vi "Connect.vi"(8 "error in (no error)":errorcluster, 9 "timeout":i32=-1, 11 "TCP Stream Listener in":refnum<class "TCP Stream Listener.lvclass">) -> (0 "error out":errorcluster, 3 "TCP Stream Listener out":refnum<class "TCP Stream Listener.lvclass">)   [LabVIEW 2020, in "TCP Stream Listener.lvclass"]
doc: "This method waits for a remote connection from a TCP/IP Stream Initiator."
uses:
  TCP Stream Listener.lvclass
  G:/Utilisateurs/hugofroylan.aragon/Documents/PyCharm/neuro/labview/Nested Endpoint Actors/Protocols/TCP Strategy/TCP Stream/TCP Stream.lvclass
  TCP Stream/TCP Stream.lvclass/TCP Stream.ctl
  TCP Stream Listener.lvclass/TCP Stream Listener.ctl
  TCP Stream/TCP Stream.lvclass
  libc.so.6
  C:/Windows/System32/ws2_32.dll
panel:
  out "return 2":i32
  out "return":i32
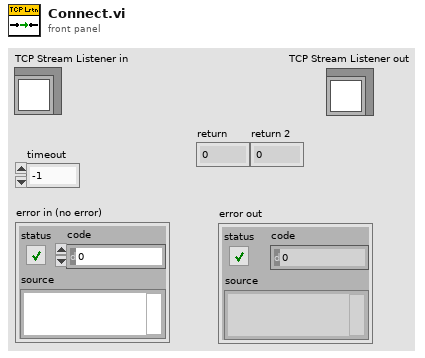
[diagram p1: front panel]
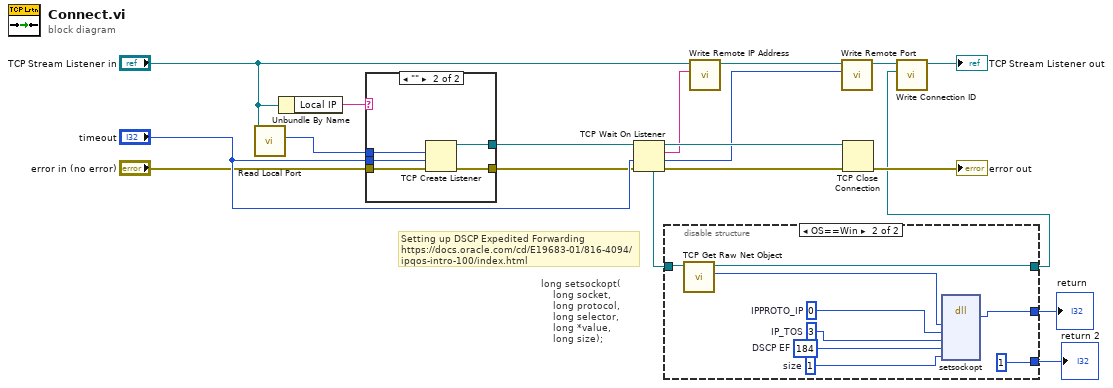
[diagram p0: block diagram]
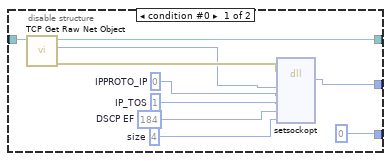
[diagram p2: hidden frame]
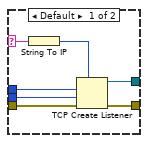
[diagram p3: hidden frame]
diagram:
  # "long setsockopt(\n    long socket,\n    long protocol,\n    long selector,\n    long *value,\n    long size);"
  # "Setting up DSCP Expedited Forwarding\nhttps://docs.oracle.com/cd/E19683-01/816-4094/ipqos-intro-100/index.html"
  n1 = call "Read Local Port.vi"("TCP Stream in"="TCP Stream Listener in") -> ("local port"=w15:u16)  [unwired: 10 in]
  n2 = Unbundle By Name("TCP Stream Listener in") -> ("Local IP"=w10:string)
  n3 = case shown="\"\"" w10 {
    selector: w10 -> [w21 _]
    tunnel: "timeout" -> [w25 w31]
    tunnel: "error in (no error)" -> [w26 w30]
    tunnel: [w22 w29] -> w5
    tunnel: [w23 w28] -> w6
    tunnel: w15 -> [w24 w27]
    frame Default {
      n4 = String To IP(1:w21) -> (0:w20:u32)
      n5 = TCP Create Listener(7:w20, 8:w26, 9:w25, 10:w24) -> (0:w22:errorcluster, 3:w23:refnum<k5>)  [unwired: 1 in, 1 out]
    }
    frame "" {
      n6 = TCP Create Listener(8:w30, 9:w31, 10:w27) -> (0:w29:errorcluster, 3:w28:refnum<k5>)  [unwired: 2 in, 1 out]
    }
  }
  n7 = TCP Wait On Listener(8:w5, 9:"timeout", 11:w6) -> (0:w7:errorcluster, 1:w11:u16, 2:w12:string, 3:w16:refnum<k5>, 4:w4:refnum<k5>)  [unwired: 1 in]
  n8 = disable-structure shown="OS==Win" {
    disable-tunnel: w4 -> [w41 w49]
    disable-tunnel: [w40 w48] -> w3
    disable-tunnel: [w33 w50] -> w2
    disable-tunnel: [0 1 ("IPPROTO_IP")] -> w1
    frame condition #0 {
      w35 = u8 184  # DSCP EF
      w36 = 4  # size
      w34 = 1  # IP_TOS
      w37 = 0  # IPPROTO_IP
      n9 = call <vilib>:"TCP Get Raw Net Object.vi"("connection ID"=w41) -> ("error out"=w39:errorcluster, "raw net object"=w38:u64, "connection ID out"=w40:refnum<k5>)  [unwired: 8 in]
      n10 = dll-call lib="libc.so.6" fn="setsockopt"(error in=w39, "sockfd"=w38, "level"=w37, "optname"=w34, "optval"=w35, "optlen"=w36) -> ("return"=w33:i32)  [unwired: 7 in, 2 out]
    }
    frame condition #1 (active) {
      w44 = u8 184  # DSCP EF
      w43 = 1  # size
      w45 = 3  # IP_TOS
      w46 = 0  # IPPROTO_IP
      n11 = call <vilib>:"TCP Get Raw Net Object.vi"("connection ID"=w49) -> ("raw net object"=w47:u64, "connection ID out"=w48:refnum<k5>)  [unwired: 8 in, 1 out]
      n12 = dll-call lib="C:/Windows/System32/ws2_32.dll" fn="setsockopt" ("Call Library Function")("socket"=w47, "protocol"=w46, "selector"=w45, "value"=w44, "size"=w43) -> ("return type"=w50:i32)  [unwired: 8 in, 2 out]
    }
  }
  "return" <- w2
  "return 2" <- w1
  n13 = call "Write Remote IP Address.vi"("Remote IP"=w12, "TCP Stream in"="TCP Stream Listener in") -> ("TCP Stream out"=w14:refnum<class "TCP Stream Listener.lvclass">)  [unwired: 9 in]
  n14 = call "Write Remote Port.vi"("remote port"=w11, "TCP Stream in"=w14) -> ("TCP Stream out"=w13:refnum<class "TCP Stream Listener.lvclass">)  [unwired: 9 in]
  n15 = TCP Close Connection(connection ID=w16, error in (no error)=w7) -> (error out=→"error out":errorcluster)  [unwired: 1 in, 1 out]
  n16 = call "Write Connection ID.vi"("connection ID"=w3, "TCP Stream in"=w13) -> ("TCP Stream out"=→"TCP Stream Listener out":refnum<class "TCP Stream Listener.lvclass">)  [unwired: 9 in]
